vi "InitEDAMessageBroker.vi"(8 "error in (no error)":errorcluster, 11 "Broker Name":string) -> (0 "error out":errorcluster, 3 "EDA Message Broker Interface Ref out":refnum<class "EDA Message Broker Interface Ref.lvclass">)   [LabVIEW 2016, in "Stream Mediator.lvlib" / "EDA Message Broker Interface Ref.lvclass"]
doc: "--\nCopyright © 2017 Composed SystemsI All rights reserved.\n\nAuthor: Jon McBee <jon.mcbee@composed.io>\n\nThis library is provided \"AS IS\" ,WITHOUT WARRANTIES OR\nCONDITIONS OF ANY KIND, either express or implied.\n\nComposed Systems -- composed.io\n\nStream 0.0.1.1\nJon McBee - Composed Systems\nCopyright (c) 2017, Composed Systems"
uses:
  <userlib>/Composed Systems/Stream/Mediator/Classes/EDA Message Broker Interface Ref/EDA Message Broker Interface Ref.lvclass
  C:/Program Files (x86)/National Instruments/LabVIEW 2016/user.lib/Composed Systems/Stream/Mediator/Classes/Message Broker Interface Ref/Message Broker Interface Ref.lvclass
  <userlib>/Composed Systems/Stream/Mediator/Classes/Topic Actor/Topic Actor.lvclass
  <userlib>/Composed Systems/Stream/Mediator/Classes/Message Broker/Message Broker.lvclass
  <userlib>/Composed Systems/Stream/Mediator/Classes/Message Broker Interface Ref/Message Broker Interface Ref.lvclass
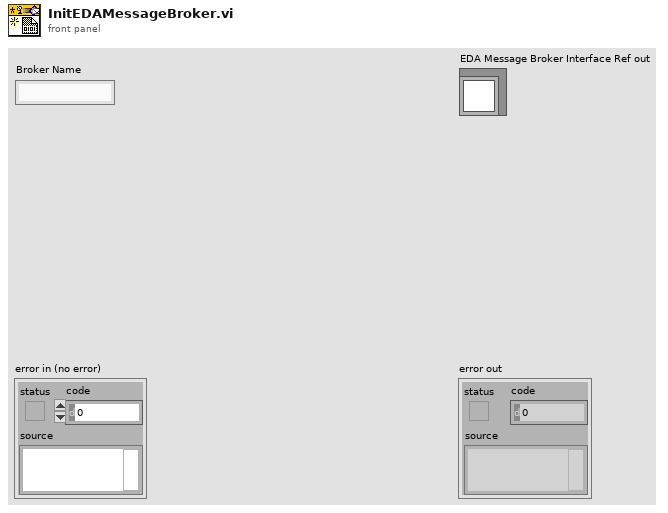
[diagram p1: front panel]
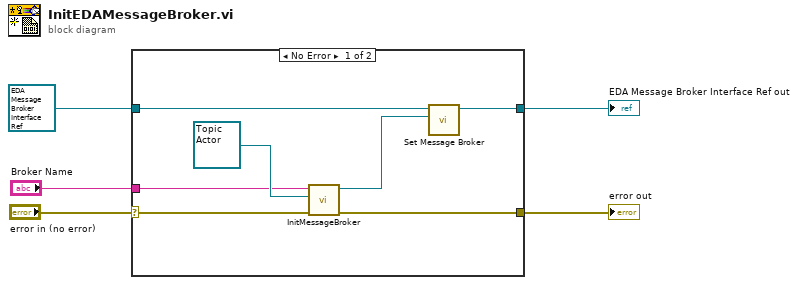
[diagram p0: block diagram]
diagram:
  n1 = case shown="No Error" "error in (no error)" {
    selector: "error in (no error)" -> [w11 w14]
    tunnel: [w10 w14] -> w4
    tunnel: [w8 w13] -> w2
    tunnel: refnum<class "EDA Message Broker Interface Ref.lvclass"> refnum ("EDA Message Broker Interface Ref in") -> [w9 w13]
    tunnel: "Broker Name" -> [w6 _]
    frame No Error {
      n2 = call <userlib>:"InitMessageBroker.vi"("error in (no error)"=w11, "Topic Actor"=refnum<class "Topic Actor.lvclass"> refnum, "Broker Name"=w6) -> ("error out"=w10:errorcluster, "Message Broker Ref"=w7:refnum<data-value>)  [unwired: 7 in]
      n3 = call <userlib>:"Set Message Broker.vi"("Broker"=w7, "Message Broker Interface Ref in"=w9) -> ("Message Broker Interface Ref out"=w8:refnum<class "EDA Message Broker Interface Ref.lvclass">)  [unwired: 8 in, 1 out]
    }
    frame Error {
    }
  }
  "error out" <- w4
  "EDA Message Broker Interface Ref out" <- w2
